vi "matchfiltering.vi"(8 "数组":cdb[](array[numeric]), 11 "簇":T1 {"簇"."pulse shaping filter" items=["none", "Raised Cosine", "Root Raised Cos", "Gsussian"]; "簇"."modulation type" items=["FSK", "PSK", "QAM", "MSK", "PAM", "ASK"]}) -> (2 "X * Y":cdb[](array[numeric]))   [LabVIEW 2014]
uses:
  <vilib>/Analysis/2dsp.llb/1D Convolution (CDB).vi
  <vilib>/addons/Modulation/Analog/support/mod_Set Error Source.vi
  <vilib>/addons/Modulation/Digital/Support/Common/Validators/mod_Generate Filter Coefficients Validate.vi
  <vilib>/addons/Modulation/Digital/General/subVIs/mod_Generate Filter Coefficients.vi
  <vilib>/addons/Modulation/niDMT.lvlib
  <vilib>/Analysis/NI_AALPro.lvlib
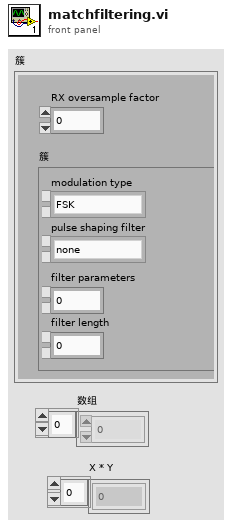
[diagram p1: front panel]
types:
  T1 = cluster{"RX oversample factor":i32, "簇":cluster{"modulation type":u16, "pulse shaping filter":u16, "filter parameters":dbl, "filter length":i32}}
  T2 = cluster{"modulation type":u16, "pulse shaping filter":u16, "filter parameters":dbl, "filter length":i32}
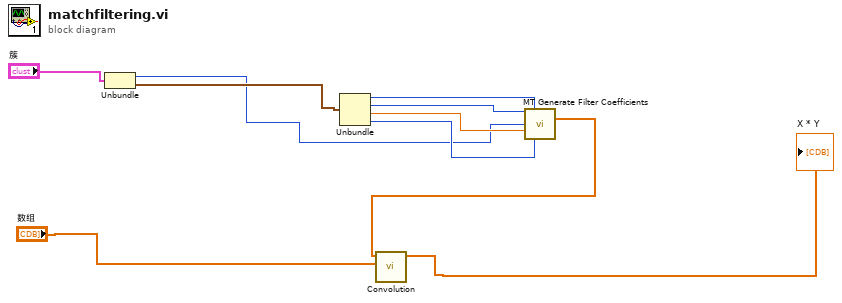
[diagram p0: block diagram]
diagram:
  n1 = Unbundle("簇") -> ("RX oversample factor"=w2:i32, "簇"=w3:T2)
  n2 = Unbundle(w3) -> ("modulation type"=w10:u16, "pulse shaping filter"=w9:u16, "filter parameters"=w8:dbl, "filter length"=w7:i32)
  n3 = call <vilib>:"MT Generate Filter Coefficients.vi"("pulse shaping filter (none)"=w9, "modulation type"=w10, "matched samples per symbol (16)"=w2, "filter parameter"=w8, "filter length (symbols)"=w7) -> ("matched filter coefficients"=w6:dbl[])  [unwired: 8 in, 2 out]
  n4 = call-poly <vilib>:"Convolution.vi"("Y"="数组", "X"=w6) -> ("X * Y"=→"X * Y":cdb[])  [unwired: 8 in, 1 out]
